vi "Request System Operator Name.vi"(8 "error in (no error)":errorcluster) -> (0 "error out":errorcluster, 2 "Operator":string)   [LabVIEW 2015]
panel:
  in  "OK Button":bool
  in  "System Operator":string
  out "Test Sequence":i32(listbox)=-2
  # "Enter System Operator"
  # "Please enter the System\nOperator Name"
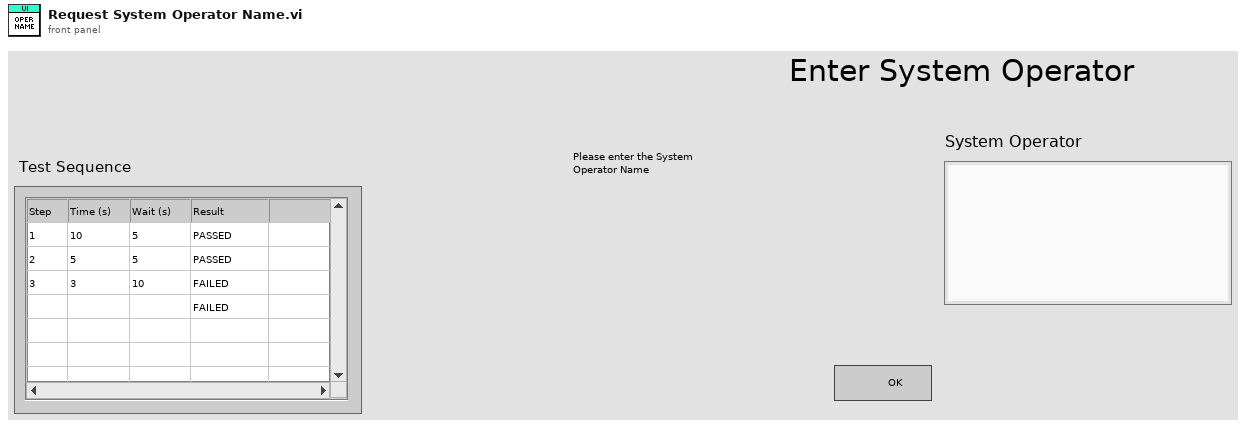
[diagram p1: front panel]
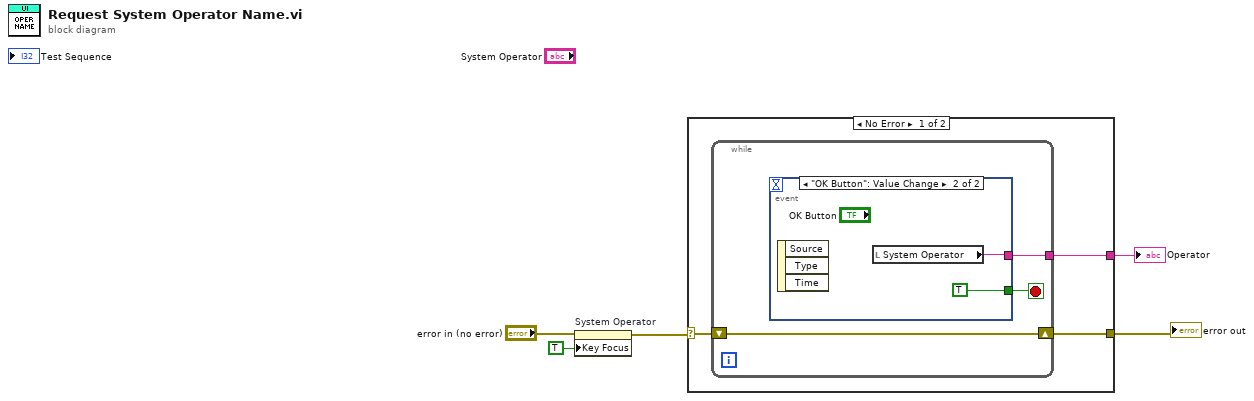
[diagram p0: block diagram]
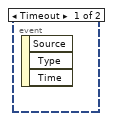
[diagram p2: hidden frame]
diagram:
  n1 = property on="System Operator" class="Str"(error in="error in (no error)", "Key Focus"=TRUE) -> (error out=w2:errorcluster)  [unwired: 1 in, 1 out]
  n2 = case shown="No Error" w2 {
    selector: w2 -> [w7 w14]
    tunnel: [w8 _] -> w5
    tunnel: [w6 w14] -> w4
    frame No Error {
      n3 = while {
        tunnel: [w10] -> w8
        shift-right: [w9] -> w6
        shift-left: w7 -> [w9]
        stop <- w11 stop-if-true
        n4 = event shown="[1] \"OK Button\": Value Change" {
          selector: _ -> [_ _]
          dyn-events: _ -> [_ _]
          timeout: _ -> [_ _]
          tunnel: [_ TRUE] -> w11
          tunnel: [_ w12] -> w10
          event Timeout {
            n5 = event-data() -> ()  [unwired: 1 in, 3 out]
          }
          event "OK Button": Value Change {
            n6 = event-data() -> ()  [unwired: 1 in, 3 out]
            n7 = local read "System Operator"() -> (w12:string)
          }
        }
      }
    }
    frame Error {
    }
  }
  "error out" <- w4
  "Operator" <- w5
